vi "Test Stand Main UI.vi"(11 "Specific Test Stand":refnum<class "Generic Test Stand.lvclass">) -> ()   [LabVIEW 2019, in "TS Framework.lvlib"]
uses:
  TS Framework.lvlib
  Generic Test Stand/Generic Test Stand.lvclass
  UI Process/UI Process Data.ctl
  ExeLogging/UI Logger/UI Logger.lvclass
  UI Process/UI State.ctl
  DAC Process/DAC Process Data.ctl
  ExeLogging/DAC Logger/DAC Logger.lvclass
  DAC Process/DAC State.ctl
  Trig Process/Trig Process Data.ctl
  Generic Test Stand/Generic Test Stand.lvclass/Generic Test Stand.ctl
  DAC Process/Exit DAC/Exit DAC.lvclass
  DAC Process/Prepare DAC Start/Prepare DAC Start.lvclass
  DAC Process/Stop DAC/Stop DAC.lvclass
  Trig Process/Stop TRIG/Stop TRIG.lvclass
  DAC Process/Save DAC Configuration/Save DAC Configuration.lvclass
  DAC Process/Select DAC Config File/Select DAC Config File.lvclass
  Trig Process/Generic Trig Command/Generic Trig Process Command.lvclass
  DAC Process/Generic DAC Command/Generic DAC Process Command.lvclass
  UI Process/Generic UI Command/Generic UI Process Command.lvclass
  UI Process/User Interface Process.lvlib
  DAC Process/DAC Process.lvlib
  Trig Process/Trig Process.lvlib
panel:
  in  "Log Details":bool=TRUE
  out "DAC Status":string caption="Data Acquisition and Control Status"
  out "Test Stand Name":string
  in  "Save Conf File":bool
  out "Config File":string
  in  "Select Config File":bool
  out "TS State":string caption="Test Stand State"
  in  "Acq Interval":dbl=1.0 caption="Acq Interval, s" min=0.5 max=3600.0 step=1.0 format="%#.1f"
  in  "Stop Acquisition":bool
  in  "Start Acquisition":bool
  in  "Exit":bool
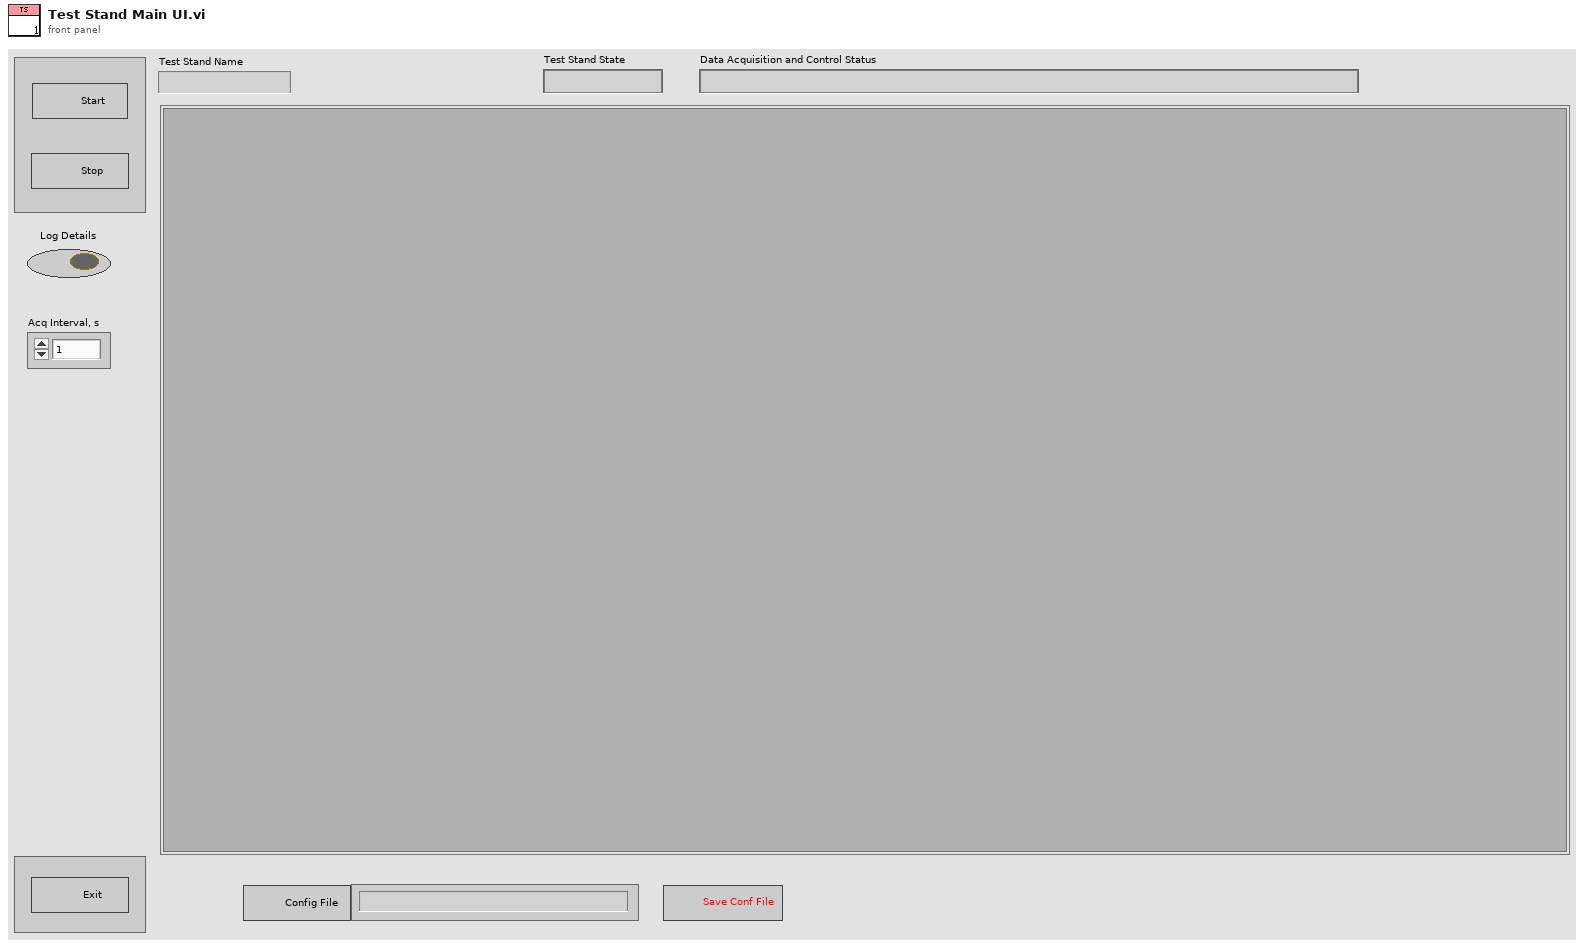
[diagram p1: front panel]
types:
  T1 = typedef "Trig Process.lvlib/Trig Process Data.ctl" = cluster{"Trig Resolution":u32, "Ctrl Interval":dbl, "Acq Interval":refnum<vi>}
  T2 = typedef "DAC Process.lvlib/DAC Process Data.ctl" = cluster{"Test Stand":refnum<class "Generic Test Stand.lvclass">, " DAC Logger":refnum<class "DAC Logger.lvclass">, "DAC State":T3, "DAC Status":refnum<vi>, "Log Details":refnum<vi>}
  T3 = typedef "DAC Process.lvlib/DAC State.ctl" = enum16{"Idle", "Acquiring"}
  T4 = typedef "User Interface Process.lvlib/UI Process Data.ctl" = cluster{"This VI":refnum<vi>, "Sub Panel Ref":refnum<vi>, "UI Logger":refnum<class "UI Logger.lvclass">, "TS Name":refnum<vi>, "Config File":refnum<vi>, "Start Acq":refnum<vi>, "Stop Acq":refnum<vi>, "Exit":refnum<vi>, "Select Conf File":refnum<vi>, "Save Conf File":refnum<vi>, "UI State":T5}
  T5 = typedef "User Interface Process.lvlib/UI State.ctl" = enum16{"Idle", "Acquiring"}
  T6 = typedef "TS Framework.lvlib/Consumer Queues.ctl" = cluster{"UI Queue":refnum<queue>, "DAC Queue":refnum<queue>, "TRIG Queue":refnum<queue>}
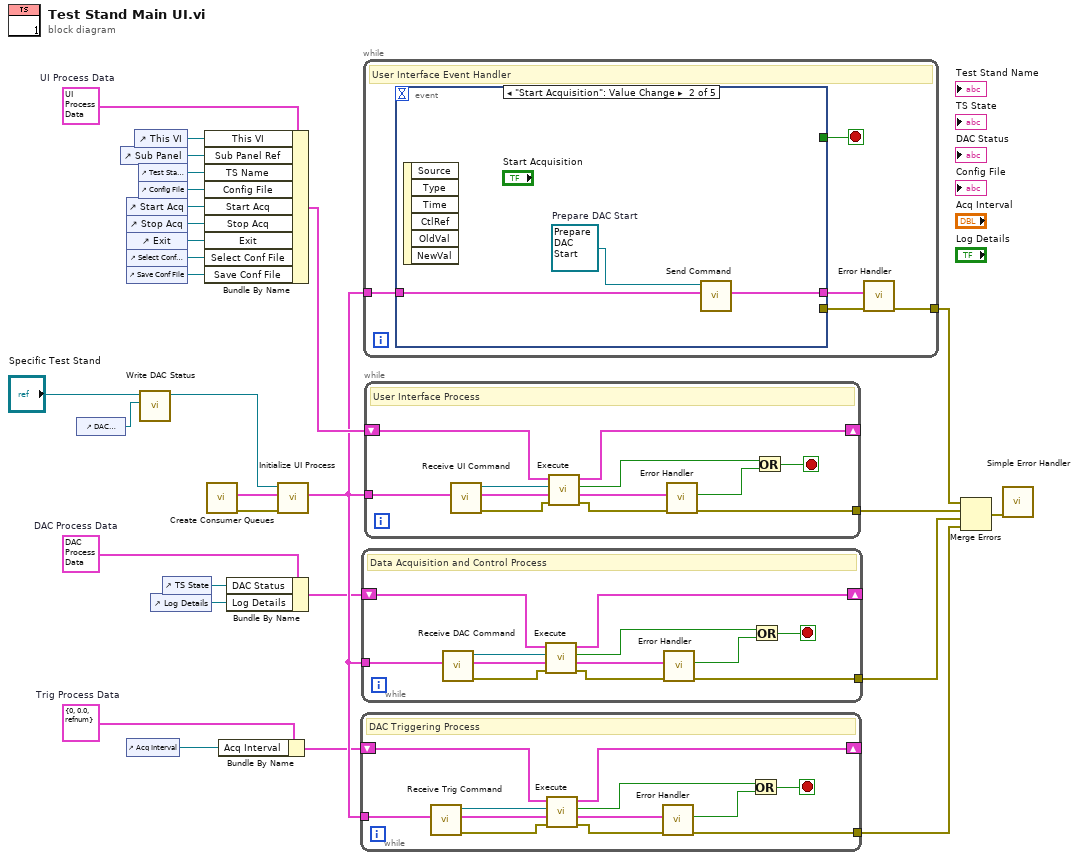
[diagram p0: block diagram]
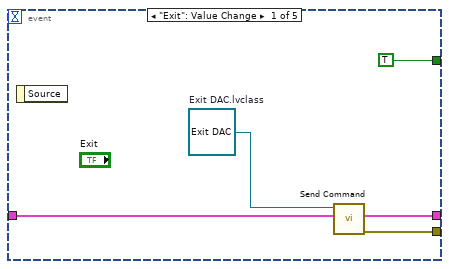
[diagram p2: hidden frame]
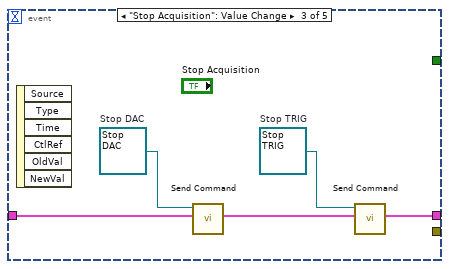
[diagram p3: hidden frame]
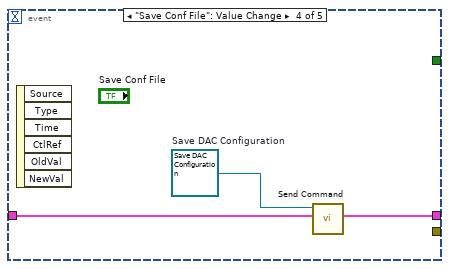
[diagram p4: hidden frame]
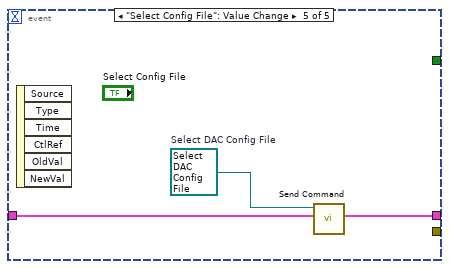
[diagram p5: hidden frame]
diagram:
  w13 = T1 {"Trig Resolution"=0, "Ctrl Interval"=0.0, "Acq Interval"=refnum}  # Trig Process Data
  w10 = T2 {"Test Stand"=refnum, " DAC Logger"=refnum, "DAC State"=enum."Idle", "DAC Status"=refnum, "Log Details"=refnum}  # DAC Process Data
  w29 = T4 {"This VI"=refnum, "Sub Panel Ref"=refnum, "UI Logger"=refnum, "TS Name"=refnum, "Config File"=refnum, "Start Acq"=refnum, "Stop Acq"=refnum, "Exit"=refnum, "Select Conf File"=refnum, "Save Conf File"=refnum, "UI State"=enum."Idle"}  # UI Process Data
  n1 = control-ref of="DAC Status"() -> (w6:refnum<vi>)
  n2 = control-ref of="Sub Panel"() -> (w25:refnum<vi>)
  n3 = control-ref of="Start Acq"() -> (w21:refnum<vi>)
  n4 = control-ref of="Stop Acq"() -> (w20:refnum<vi>)
  n5 = control-ref of="Exit"() -> (w19:refnum<vi>)
  n6 = control-ref of="Select Conf File"() -> (w18:refnum<vi>)
  n7 = control-ref of="Save Conf File"() -> (w17:refnum<vi>)
  n8 = control-ref of="Acq Interval"() -> (w2:refnum<vi>)
  n9 = control-ref of="This VI"() -> (w28:refnum<vi>)
  n10 = control-ref of="Test Stand Name"() -> (w23:refnum<vi>)
  n11 = control-ref of="Config File"() -> (w22:refnum<vi>)
  n12 = call "Write DAC Status.vi"("DAC Status"=w6, "Generic Test Stand in"="Specific Test Stand") -> ("Generic Test Stand out"=w4:refnum<class "Generic Test Stand.lvclass">)  [unwired: 8 in, 1 out]
  n13 = control-ref of="Log Details"() -> (w1:refnum<vi>)
  n14 = control-ref of="TS State"() -> (w8:refnum<vi>)
  n15 = Bundle By Name(cluster=w29, "This VI"=w28, "Sub Panel Ref"=w25, "TS Name"=w23, "Config File"=w22, "Start Acq"=w21, "Stop Acq"=w20, "Exit"=w19, "Select Conf File"=w18, "Save Conf File"=w17) -> (w27:T4)
  n16 = call "Create Consumer Queues.vi"() -> ("error out"=w5:errorcluster, "Consumer Queues"=w24:T6)  [unwired: 10 in]
  n17 = Bundle By Name(cluster=w13, "Acq Interval"=w2) -> (w3:T1)
  n18 = Bundle By Name(cluster=w10, "DAC Status"=w8, "Log Details"=w1) -> (w9:T2)
  n19 = call "Initialize UI Process.vi"("error in (no error)"=w5, "Consumer Queues in"=w24, "Test Stand.lvclass"=w4) -> ("Consumer Queues out"=w16:T6)  [unwired: 7 in, 1 out]
  n20 = while {
    shift-right: [w36] -> _
    shift-left: w3 -> [w37]
    tunnel: w16 -> [w38]
    tunnel: [w39] -> w14
    stop <- w40 stop-if-true
    # "DAC Triggering Process"
    n21 = call "Receive Trig Command.vi"("Consumer Queues in"=w38) -> ("error out"=w33:errorcluster, "Consumer Queues out"=w34:T6, "Trig Process Command out"=w35:refnum<class "Generic Trig Process Command.lvclass">)  [unwired: 8 in]
    n22 = call-dynamic "Execute.vi"("error in (no error)"=w33, "Consumer Queues in"=w34, "Trig Process Command in"=w35, "Trig Process Data in"=w37) -> ("error out"=w30:errorcluster, "Consumer Queues out"=w31:T6, "Stop?"=w32:bool, "Trig Process Data out"=w36:T1)  [unwired: 4 in]
    n23 = call "Error Handler.vi"("error in (no error)"=w30, "Consumer Queues in"=w31) -> ("error out"=w39:errorcluster, "Stop?"=w41:bool)  [unwired: 8 in]
    n24 = Or(x=w32, y=w41) -> (x .or. y?=w40:bool)
  }
  n25 = while {
    shift-right: [w50] -> _
    shift-left: w9 -> [w51]
    tunnel: w16 -> [w43]
    tunnel: [w42] -> w15
    stop <- w44 stop-if-true
    # "Data Acquisition and Control Process"
    n26 = call "Receive DAC Command.vi"("Consumer Queues in"=w43) -> ("error out"=w52:errorcluster, "Consumer Queues out"=w49:T6, "DAC Process Command out"=w53:refnum<class "Generic DAC Process Command.lvclass">)  [unwired: 8 in]
    n27 = call-dynamic "Execute.vi"("error in"=w52, "Consumer Queues in"=w49, "DAC Process Command in"=w53, "DAC Process Data in"=w51) -> ("error out"=w47:errorcluster, "Consumer Queues out"=w48:T6, "Stop?"=w46:bool, "DAC Process Data out"=w50:T2)  [unwired: 4 in]
    n28 = call "Error Handler.vi"("error in (no error)"=w47, "Consumer Queues in"=w48) -> ("error out"=w42:errorcluster, "Stop?"=w45:bool)  [unwired: 8 in]
    n29 = Or(x=w46, y=w45) -> (x .or. y?=w44:bool)
  }
  n30 = while {
    tunnel: w16 -> [w55]
    tunnel: [w54] -> w11
    stop <- w58 stop-if-true
    # "User Interface Event Handler"
    n31 = event shown="[1] \"Start Acquisition\": Value Change" {
      selector: _ -> [_ _ _ _ _]
      dyn-events: _ -> [_ _ _ _ _]
      timeout: _ -> [_ _ _ _ _]
      tunnel: [w63 w65 w68 w73 w76] -> w57
      tunnel: [TRUE _ _ _ _] -> w58
      tunnel: [w61 _ _ _ _] -> w56
      tunnel: w55 -> [w60 w66 w71 w74 w77]
      event "Exit": Value Change {
        w59 = refnum<class "Exit DAC.lvclass"> refnum  # Exit DAC.lvclass
        n32 = event-data() -> ()  [unwired: 1 in, 1 out]
        n33 = call-dynamic "Send Command.vi"("Consumer Queues in"=w60, "DAC Process Command"=w59) -> ("error out"=w61:errorcluster, "Consumer Queues out"=w63:T6)  [unwired: 8 in]
      }
      event "Start Acquisition": Value Change {
        w64 = refnum<class "Prepare DAC Start.lvclass"> refnum  # Prepare DAC Start
        n34 = event-data() -> ()  [unwired: 1 in, 6 out]
        n35 = call-dynamic "Send Command.vi"("Consumer Queues in"=w66, "DAC Process Command"=w64) -> ("Consumer Queues out"=w65:T6)  [unwired: 8 in, 1 out]
      }
      event "Stop Acquisition": Value Change {
        w67 = refnum<class "Stop TRIG.lvclass"> refnum  # Stop TRIG
        w70 = refnum<class "Stop DAC.lvclass"> refnum  # Stop DAC
        n36 = event-data() -> ()  [unwired: 1 in, 6 out]
        n37 = call-dynamic "Send Command.vi"("Consumer Queues in"=w71, "DAC Process Command"=w70) -> ("Consumer Queues out"=w69:T6)  [unwired: 8 in, 1 out]
        n38 = call-dynamic "Send Command.vi"("Consumer Queues in"=w69, "Trig Process Command"=w67) -> ("Consumer Queues out"=w68:T6)  [unwired: 8 in, 1 out]
      }
      event "Save Conf File": Value Change {
        w72 = refnum<class "Save DAC Configuration.lvclass"> refnum  # Save DAC Configuration
        n39 = event-data() -> ()  [unwired: 1 in, 6 out]
        n40 = call-dynamic "Send Command.vi"("Consumer Queues in"=w74, "DAC Process Command"=w72) -> ("Consumer Queues out"=w73:T6)  [unwired: 8 in, 1 out]
      }
      event "Select Config File": Value Change {
        w75 = refnum<class "Select DAC Config File.lvclass"> refnum  # Select DAC Config File
        n41 = event-data() -> ()  [unwired: 1 in, 6 out]
        n42 = call-dynamic "Send Command.vi"("Consumer Queues in"=w77, "DAC Process Command"=w75) -> ("Consumer Queues out"=w76:T6)  [unwired: 8 in, 1 out]
      }
    }
    n43 = call "Error Handler.vi"("error in (no error)"=w56, "Consumer Queues in"=w57) -> ("error out"=w54:errorcluster)  [unwired: 8 in, 1 out]
  }
  n44 = while {
    shift-right: [w87] -> _
    shift-left: w27 -> [w88]
    tunnel: [w82] -> w12
    tunnel: w16 -> [w78]
    stop <- w79 stop-if-true
    # "User Interface Process"
    n45 = call "Receive UI Command.vi"("Consumer Queues in"=w78) -> ("error out"=w86:errorcluster, "Consumer Queues out"=w85:T6, "UI Process Command out"=w89:refnum<class "Generic UI Process Command.lvclass">)  [unwired: 8 in]
    n46 = call-dynamic "Execute.vi"("error in (no error)"=w86, "Consumer Queues in"=w85, "UI Process Command in"=w89, "UI Process Data in"=w88) -> ("error out"=w84:errorcluster, "Consumer Queues out"=w83:T6, "Stop?"=w80:bool, "UI Process Data out"=w87:T4)  [unwired: 4 in]
    n47 = call "Error Handler.vi"("error in (no error)"=w84, "Consumer Queues in"=w83) -> ("error out"=w82:errorcluster, "Stop?"=w81:bool)  [unwired: 8 in]
    n48 = Or(x=w80, y=w81) -> (x .or. y?=w79:bool)
  }
  n49 = Merge Errors(w11, w12, w15, w14) -> (w26:errorcluster)
  n50 = call <vilib>:"Simple Error Handler.vi"("error in (no error)"=w26) -> ()  [unwired: 4 in, 5 out]
